vi "Read Data.vi"() -> ()   [LabVIEW 2015]
panel:
  in  "stop":bool
  out "Data Chart":dbl(graph)
  in  "Time Delay (ms)":u32(slide) scale=0.0..200.0
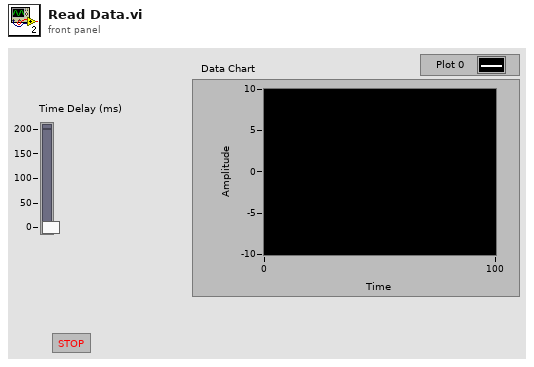
[diagram p1: front panel]
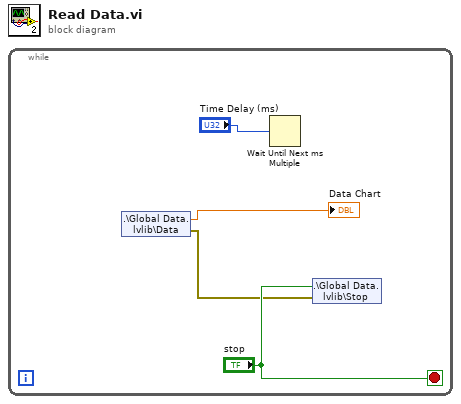
[diagram p0: block diagram]
diagram:
  n1 = while {
    stop <- "stop" stop-if-true
    n2 = shared-variable ".\\Global Data.lvlib\\Data"() -> (→"Data Chart":dbl, error out=w1:errorcluster)  [unwired: 1 in]
    n3 = Wait Until Next ms Multiple(millisecond multiple="Time Delay (ms)") -> ()  [unwired: 1 out]
    n4 = shared-variable ".\\Global Data.lvlib\\Stop"("stop", error in=w1) -> ()  [unwired: 1 out]
  }
